vi "Cfg List _ Update Channel List.vi"(7 "ColInfo":T1, 8 "错误输入":errorcluster caption="错误输入（无错误）", 10 "ModuCfg":T2, 11 "TreeRef":refnum<vi>) -> (0 "错误输出":errorcluster, 2 "ColHeaders[]":string[](array[string]))   [LabVIEW 2016]
uses:
  HardWare/Ctrls/HardWare _ Module Configuration.ctl
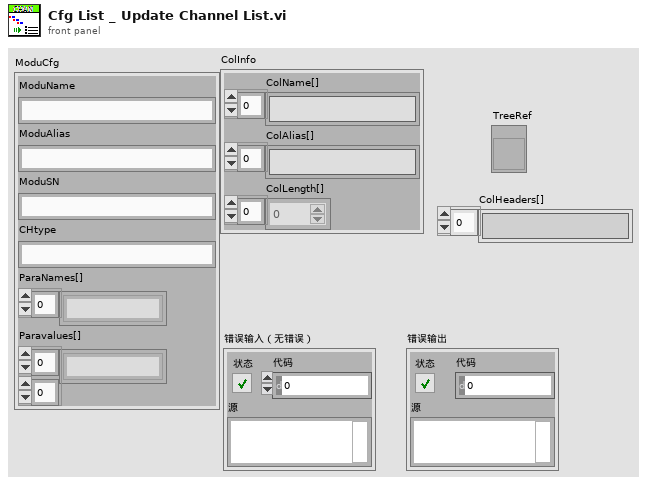
[diagram p1: front panel]
types:
  T1 = cluster{"ColName[]":string[], "ColAlias[]":string[], "ColLength[]":i32[]}
  T2 = typedef "HardWare _ Module Configuration.ctl" = cluster{"ModuName":string, "ModuAlias":string, "ModuSN":string, "CHtype":string, "ParaNames[]":string[], "Paravalues[]":string[][]}
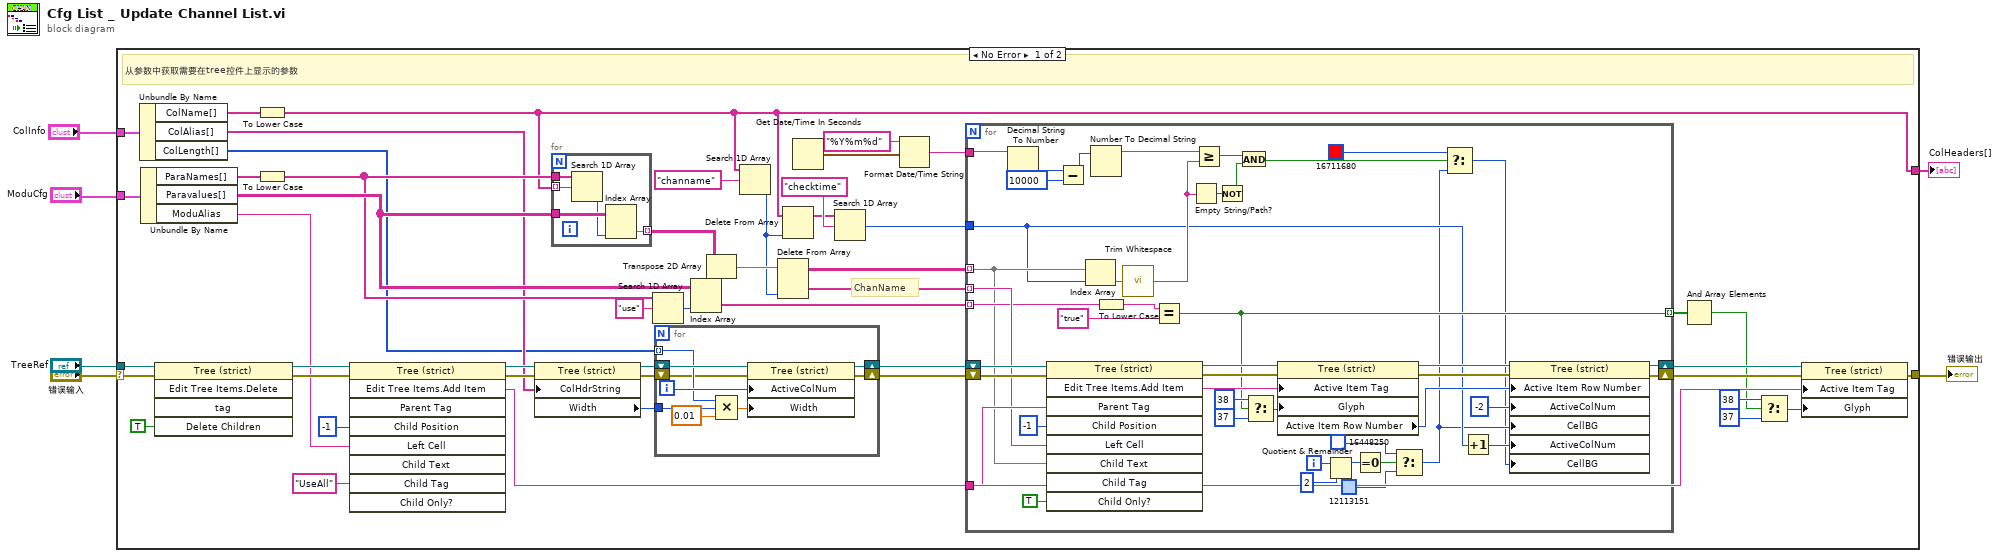
[diagram p0: block diagram]
diagram:
  n1 = case shown="No Error" "错误输入" {
    selector: "错误输入" -> [w52 w113]
    tunnel: "TreeRef" -> [w53 _]
    tunnel: [w36 w113] -> w5
    tunnel: "ModuCfg" -> [w51 _]
    tunnel: [w13 _] -> w2
    tunnel: "ColInfo" -> [w23 _]
    frame No Error {
      # "ChanName"
      # "从参数中获取需要在tree控件上显示的参数"
      n2 = Unbundle By Name(w23) -> ("ColName[]"=w21:string[], "ColAlias[]"=w22:string[], "ColLength[]"=w18:i32[])
      n3 = Unbundle By Name(w51) -> ("ParaNames[]"=w28:string[], "Paravalues[]"=w27:string[][], "ModuAlias"=w29:string)
      n4 = invoke class="Tree (strict)" method="Edit Tree Items.Delete"(reference=w53, error in=w52, "Delete Children"=TRUE ("删除子项？")) -> (reference out=w49:refnum<vi>, error out=w48:errorcluster)  [unwired: 2 in, 3 out]
      n5 = To Lower Case(string=w21) -> (all lower case string=w13:string[])
      n6 = To Lower Case(string=w28) -> (all lower case string=w24:string[])
      n7 = invoke class="Tree (strict)" method="Edit Tree Items.Add Item"(reference=w49, error in=w48, "Child Position"=-1 ("子项位置"), "Left Cell"=w29, "Child Tag"="UseAll" ("子项标识符")) -> (reference out=w40:refnum<vi>, error out=w39:errorcluster, "Edit Tree Items:Add Item"=w35:string)  [unwired: 4 in, 6 out]
      n8 = property class="Tree (strict)"(reference=w40, error in=w39, "ColHdrString"=w22) -> (reference out=w20:refnum<vi>, error out=w17:errorcluster, "Width"=w19:u32)
      n9 = for {
        tunnel: w13 -> [w63] mode=indexing
        tunnel: w24 -> [w67]
        tunnel: w27 -> [w66]
        tunnel: [w64] -> w14 mode=indexing
        n10 = Search 1D Array(1D array=w67, element=w63) -> (index of element=w65:i32)  [unwired: 1 in]
        n11 = Index Array(array=w66, index (col)=w65) -> (element=w64:string[])  [unwired: 1 in]
      }
      n12 = Search 1D Array(1D array=w24, element="use" ("元素")) -> (index of element=w25:i32)  [unwired: 1 in]
      n13 = for {
        shift-right: [w56] -> _
        shift-left: w20 -> [w62]
        tunnel: w19 -> [w58]
        tunnel: w18 -> [w59] mode=indexing
        shift-right: [w54] -> w16
        shift-left: w17 -> [w55]
        i -> [w61]
        n14 = Compound Arithmetic op=MULTIPLY(w59, w58, 0.01) -> (w60:dbl)
        n15 = property class="Tree (strict)"(reference=w62, error in=w55, "ActiveColNum"=w61, "Width"=w60) -> (reference out=w56:refnum<vi>, error out=w54:errorcluster)
      }
      n16 = Index Array(array=w27, index (col)=w25) -> (element=w44:string[])  [unwired: 1 in]
      n17 = Transpose 2D Array(2D array=w14) -> (transposed array=w26:string[][])
      n18 = Search 1D Array(1D array=w13, element="channame" ("元素")) -> (index of element=w12:i32)  [unwired: 1 in]
      n19 = Delete From Array(array=w26, index (col)=w12) -> (deleted portion=w42:string[], array with subset deleted=w41:string[][])  [unwired: 2 in]
      n20 = Delete From Array(array=w13, index=w12) -> (array with subset deleted=w11:string[])  [unwired: 1 in, 1 out]
      n21 = Get Date/Time In Seconds() -> (seconds since 1Jan1904=w9:timestamp)
      n22 = Search 1D Array(1D array=w11, element="checktime" ("元素")) -> (index of element=w10:i32)  [unwired: 1 in]
      n23 = Format Date/Time String(time format string (%c)="%Y%m%d", seconds (now)=w9) -> (date/time string=w7:string)  [unwired: 1 in]
      n24 = for {
        shift-right: [w88] -> w38
        shift-left: w20 -> [w112]
        shift-right: [w87] -> w37
        shift-left: w16 -> [w111]
        tunnel: w44 -> [w104] mode=indexing
        tunnel: w42 -> [w108] mode=indexing
        tunnel: w41 -> [w84] mode=indexing
        tunnel: w35 -> [w110]
        tunnel: [w98] -> w34 mode=indexing
        tunnel: w10 -> [w79]
        tunnel: w7 -> [w72]
        i -> [w96]
        n25 = Decimal String To Number(string=w72) -> (number=w71:i32)  [unwired: 2 in, 1 out]
        n26 = invoke class="Tree (strict)" method="Edit Tree Items.Add Item"(reference=w112, error in=w111, "Parent Tag"=w110, "Child Position"=-1 ("子项位置"), "Left Cell"=w108, "Child Text"=w84, "Child Only?"=TRUE) -> (reference out=w107:refnum<vi>, error out=w106:errorcluster, "Edit Tree Items:Add Item"=w105:string)  [unwired: 2 in, 6 out]
        n27 = Subtract(x=w71, y=10000) -> (x-y=w69:i32)
        n28 = Index Array(array=w84, index=w79) -> (element=w83:string)
        n29 = Number To Decimal String(number=w69) -> (decimal integer string=w68:string)  [unwired: 1 in]
        n30 = To Lower Case(string=w104) -> (all lower case string=w103:string)
        n31 = call <vilib>:"Trim Whitespace.vi"("string"=w83) -> ("trimmed string"=w81:string)  [unwired: 1 in]
        n32 = Equal?(x=w103, y="true") -> (x = y?=w98:bool)
        n33 = Empty String/Path?(string/path=w81) -> (empty?=w80:bool)
        n34 = Greater Or Equal?(x=w68, y=w81) -> (x >= y?=w82:bool)
        n35 = Not(x=w80) -> (.not. x?=w73:bool)
        n36 = And(x=w82, y=w73) -> (x .and. y?=w77:bool)
        n37 = Select(t=38 ("活动项:符号索引"), s=w98, f=37 ("活动项:符号索引")) -> (s? t:f=w100:i32)
        n38 = property class="Tree (strict)"(reference=w107, error in=w106, "Active Item Tag"=w105, "Glyph"=w100) -> (reference out=w90:refnum<vi>, error out=w89:errorcluster, "Active Item Row Number"=w86:i32)
        n39 = Quotient & Remainder(x=w96, y=2) -> (x-y*floor(x/y)=w94:i32)  [unwired: 1 out]
        n40 = Equal To 0?(x=w94) -> (x = 0?=w93:bool)
        n41 = Select(t=u32 16448250, s=w93, f=u32 12113151) -> (s? t:f=w75:u32)
        n42 = Select(t=u32 16711680, s=w77, f=w75) -> (s? t:f=w74:u32)
        n43 = Increment(x=w79) -> (x+1=w78:i32)
        n44 = property class="Tree (strict)"(reference=w90, error in=w89, "Active Item Row Number"=w86, "ActiveColNum"=-2 ("Active Cell:Active Column Number"), "CellBG"=w75, "ActiveColNum"=w78, "CellBG"=w74) -> (reference out=w88:refnum<vi>, error out=w87:errorcluster)
      }
      n45 = And Array Elements(Boolean array=w34) -> (logical AND=w30:bool)
      n46 = Select(t=38 ("活动项:符号索引"), s=w30, f=37 ("活动项:符号索引")) -> (s? t:f=w31:i32)
      n47 = property class="Tree (strict)"(reference=w38, error in=w37, "Active Item Tag"=w35, "Glyph"=w31) -> (error out=w36:errorcluster)  [unwired: 1 out]
    }
    frame Error {
    }
  }
  "错误输出" <- w5
  "ColHeaders[]" <- w2
